vi "Refresh Groups Table.vi"(8 "error in (no error)":errorcluster, 9 "Index":i32=-1, 10 "MulticolumnListbox in":refnum<vi>, 11 "Item Ref in":T1 format="%.0x") -> (0 "error out":errorcluster, 2 "Array":string[][](array[string]), 3 "Item Ref out":T1 format="%.0x")   [LabVIEW 2027, in "Embedded Data Logger System Explorer.lvlib"]
uses:
  Embedded Data Logger System Explorer.lvlib
  <vilib>/NI VeriStand/Custom Device API/Custom Device Item Ref.ctl
  <vilib>/NI VeriStand/Custom Device API/Custom Device API.lvlib
  Scripting/Embedded Data Logger Scripting.lvlib
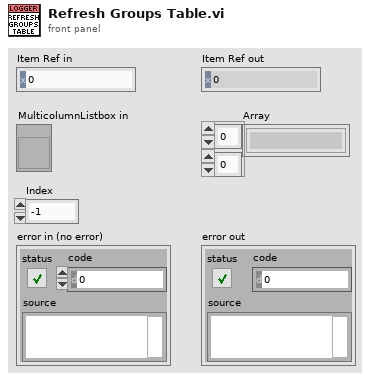
[diagram p1: front panel]
types:
  T1 = typedef "Custom Device API.lvlib/Custom Device Item Ref.ctl" = u64
  T2 = typedef "Custom Device API.lvlib/Custom Device Item Info.ctl" = cluster{"Name":string, "Is Channel":bool, "GUID":string, "Is Waveform":bool}
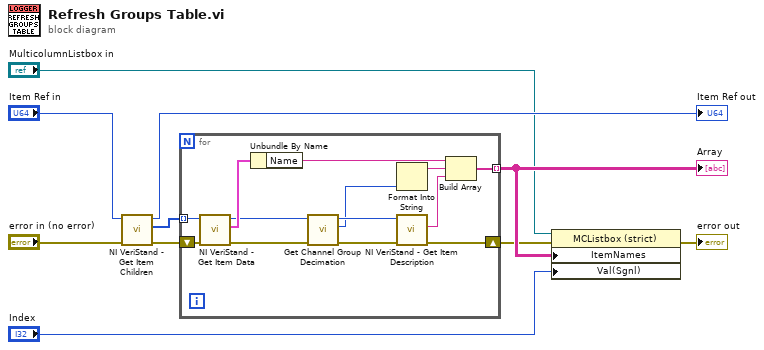
[diagram p0: block diagram]
diagram:
  n1 = call <vilib>:"NI VeriStand - Get Item Children.vi"("error in (no error)"="error in (no error)", "Item Ref in"="Item Ref in") -> ("error out"=w6:errorcluster, "Child Refs"=w7:T1[], "Item Ref out"=→"Item Ref out":T1)  [unwired: 6 in, 1 out]
  n2 = for {
    tunnel: w7 -> [w22] mode=indexing
    tunnel: [w17] -> w10 mode=indexing
    shift-right: [w16] -> w2
    shift-left: w6 -> [w23]
    n3 = call <vilib>:"NI VeriStand - Get Item Data.vi"("error in (no error)"=w23, "Item Ref in"=w22) -> ("error out"=w15:errorcluster, "Item Info"=w21:T2, "Item Ref out"=w14:T1)  [unwired: 6 in, 1 out]
    n4 = Unbundle By Name(w21) -> ("Name"=w20:string)
    n5 = call "Get Channel Group Decimation.vi"("error in"=w15, "channel group in"=w14) -> ("error out"=w13:errorcluster, "decimation"=w11:i32, "channel group out"=w12:T1)  [unwired: 7 in]
    n6 = Format Into String(w11) -> (resulting string=w19:string)  [unwired: 3 in, 1 out]
    n7 = call <vilib>:"NI VeriStand - Get Item Description.vi"("error in (no error)"=w13, "Item Ref in"=w12) -> ("error out"=w16:errorcluster, "Description"=w18:string)  [unwired: 6 in, 2 out]
    n8 = Build Array(w20, w19, w18) -> (w17:string[])
  }
  "Array" <- w10
  n9 = property on="Property Node" class="MCListbox (strict)"(reference="MulticolumnListbox in", error in=w2, "ItemNames"=w10, "Val(Sgnl)"="Index") -> (error out=→"error out":errorcluster)  [unwired: 1 out]
